vi "GEOM_BinDetStruct.vi"(10 "GEOM_FPAReadModes":T1[](array[typedef]) {"Amplifiers"."fliped" items=["none", "horizontal", "vertical"]; "Amplifiers"."type" items=["LL", "LR", "UL", "UR"]}) -> ()   [LabVIEW 2016]
uses:
  GEOM_FPAReadMode.ctl
  GEOM_Amplifier.ctl
  GEOM_AmpType.ctl
  GEOM_ROI.ctl
  GEOM_Coords.ctl
  GEOM_VAR_action.ctl
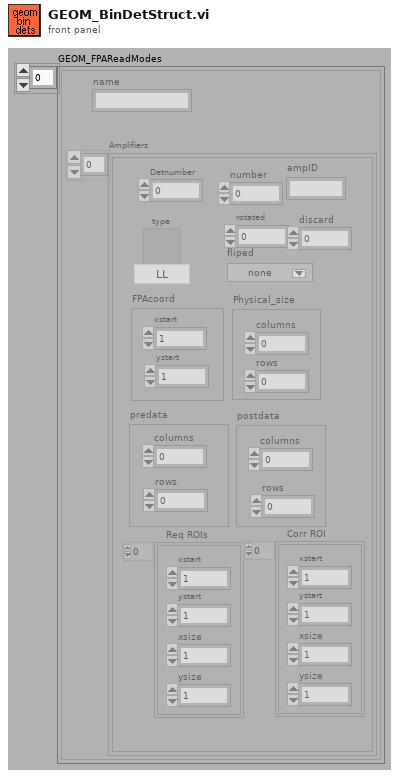
[diagram p1: front panel]
types:
  T1 = typedef "GEOM_FPAReadMode.ctl" = cluster{"name":string, "Amplifiers":T2[]}
  T2 = typedef "GEOM_Amplifier.ctl" = cluster{"number":i32, "type":T3, "rotated":i16, "fliped":u16, "FPAcoord":cluster{"xstart":i32, "ystart":i32}, "Physical_size":cluster{"columns":i32, "rows":i32}, "predata":cluster{"columns":i32, "rows":i32}, "postdata":cluster{"columns":i32, "rows":i32}, "Req ROIs":T4, "Corr ROI":T4, "Detnumber":i32, "ampID":string, "discard":i32}
  T3 = typedef "GEOM_AmpType.ctl" = u16
  T4 = typedef "GEOM_ROI.ctl" = T5[]
  T5 = typedef "GEOM_Coords.ctl" = cluster{"xstart":u32, "ystart":u32, "xsize":u32, "ysize":u32}
  T6 = typedef "GEOM_VAR_action.ctl" = enum16{"read", "write"}
  T7 = typedef "GEOM_DetSummaryStruct.ctl" = cluster{"detxpos":i32, "detypos":i32, "cols":i32, "rows":i32, "nxamps":i32, "nyamps":i32, "number":i32, "discard":i32, "totcols":i32, "totrows":i32, "readmode":string}
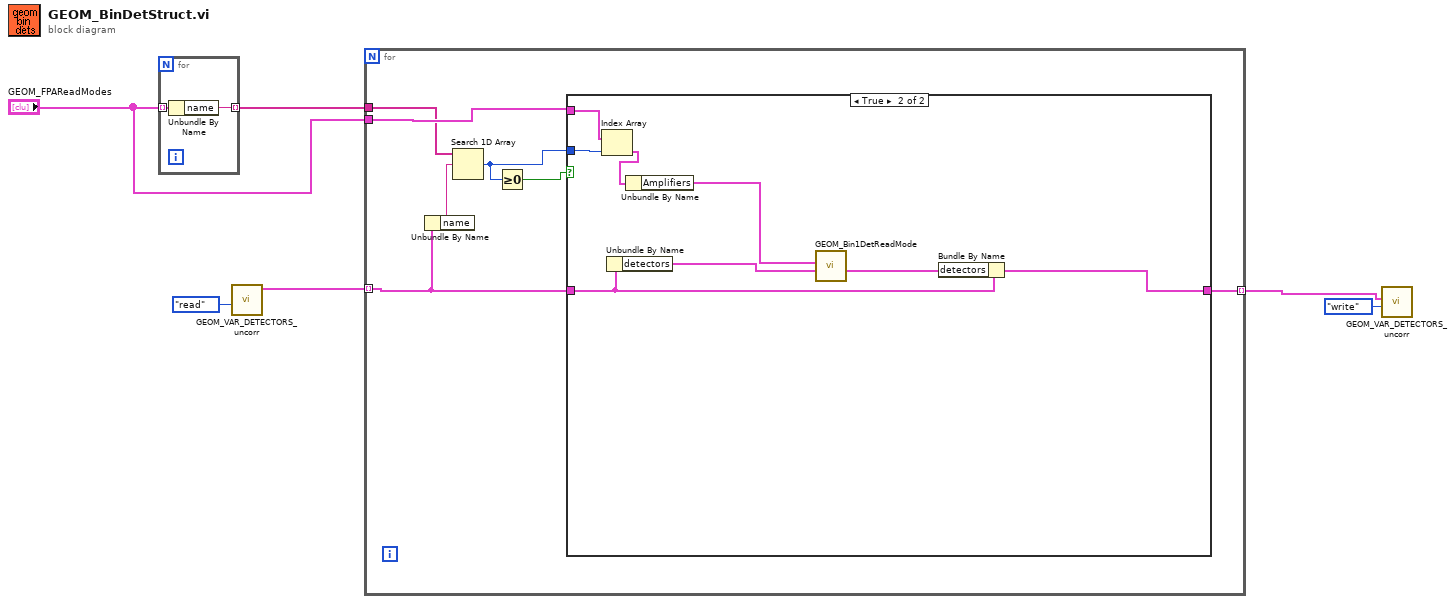
[diagram p0: block diagram]
diagram:
  n1 = for {
    tunnel: "GEOM_FPAReadModes" -> [w8] mode=indexing
    tunnel: [w7] -> w5 mode=indexing
    n2 = Unbundle By Name(w8) -> ("name"=w7:string)
  }
  n3 = call "GEOM_VAR_DETECTORS_uncorr.vi"("Action"=GEOM_VAR_action."read") -> ("det out"=w1:cluster{"name":string, "detectors":T7[]}[])  [unwired: 1 in, 9 out]
  n4 = for {
    tunnel: "GEOM_FPAReadModes" -> [w15]
    tunnel: w1 -> [w13] mode=indexing
    tunnel: [w14] -> w4 mode=indexing
    tunnel: w5 -> [w12]
    n5 = Unbundle By Name(w13) -> ("name"=w9:string)
    n6 = Search 1D Array(1D array=w12, element=w9) -> (index of element=w10:i32)  [unwired: 1 out]
    n7 = Greater Or Equal To 0?(x=w10) -> (x >= 0?=w11:bool)
    n8 = case shown="True" w11 {
      tunnel: w15 -> [_ w24]
      tunnel: [w16 w17] -> w14
      tunnel: w13 -> [w16 w19]
      tunnel: w10 -> [_ w23]
      frame False {
      }
      frame True {
        n9 = Index Array(array=w24, index=w23) -> (element=w22:T1)
        n10 = Unbundle By Name(w19) -> ("detectors"=w20:T7[])
        n11 = Unbundle By Name(w22) -> ("Amplifiers"=w21:T2[])
        n12 = call "GEOM_Bin1DetReadMode.vi"("detectors"=w20, "Amplifiers"=w21) -> ("detectors out"=w18:T7[])  [unwired: 9 out]
        n13 = Bundle By Name(cluster=w19, "detectors"=w18) -> (w17:cluster{"name":string, "detectors":T7[]})
      }
    }
  }
  n14 = call "GEOM_VAR_DETECTORS_uncorr.vi"("Action"=GEOM_VAR_action."write", "det in"=w4) -> ()  [unwired: 10 out]
